vi "util_equal_column_width.vi"(11 "Input 1D array":string[](array[string])) -> (3 "Output 1D array":string[](array[string]))   [LabVIEW 2016]
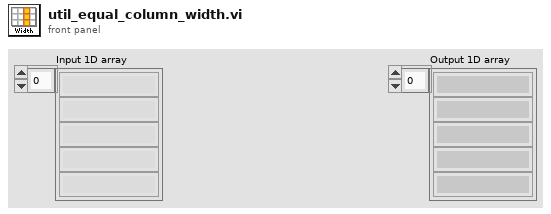
[diagram p1: front panel]
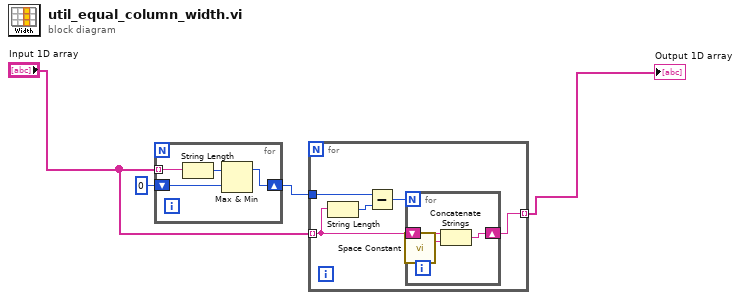
[diagram p0: block diagram]
diagram:
  n1 = for {
    tunnel: "Input 1D array" -> [w8] mode=indexing
    shift-right: [w5] -> w3
    shift-left: 0 -> [w6]
    n2 = String Length(string=w8) -> (length=w7:i32)
    n3 = Max & Min(x=w7, y=w6) -> (max(x,y)=w5:i32)  [unwired: 1 out]
  }
  n4 = for {
    tunnel: "Input 1D array" -> [w10] mode=indexing
    tunnel: w3 -> [w12]
    tunnel: [w9] -> w1 mode=indexing
    n5 = String Length(string=w10) -> (length=w13:i32)
    n6 = Subtract(x=w12, y=w13) -> (x-y=w11:i32)
    n7 = for {
      N: w11 -> [_]
      shift-right: [w16] -> w9
      shift-left: w10 -> [w15]
      n8 = call <vilib>:"Space Constant.vi"() -> ("String"=w14:string)
      n9 = Concatenate Strings(w15, w14) -> (w16:string)
    }
  }
  "Output 1D array" <- w1
